vi "FRA-GRAPHs.vi"() -> ()   [LabVIEW 2014]
panel:
  in  "Waveform Graph":dbl[][](graph)=[[755.8497899944483, 657.3694630192037, 604.2075862163476, 553.4051094764117, 501.397888353343, 457.9831143953616, 522.5385383457407, 449.43840743756704, 491.0669063418323, 427.9053041861322, 472.8329741058286, 734.0752884613231, 754.8685930222813, 867.8139215972071, 764.1663113926469, 1052.3750959044867, 370.47956063576765, -5454.671583974405, 5956.812472120322, 3291.774216244163, 2978.0635239759176, 24470.64307332704, 24011.616955981375, 4002.6341189398554, 10685.523439025172, -1848.0447542106147, -644.1201502824483, 14733.80660145546, 35622.61812955256, 14965.266379348848, -30861.486423716706, 1459.6554322016723, -3196.3540839642674, 44188.99982358876, 45267.97553031476, 142706.1244173352, 53308.369203099464, -27391.526865018615, 183165.8872198102, -87308.9518464976, -120174.13920583515, 26604.096776415798, -493090.5307564318, 366117.10634527745, 543287.8874074903, -2290216.410117346, 1383746.3098287373, -841011.6581585368, -5069703.915509953], [12809.615219888727, 14640.640733060218, 16941.76975803665, 19632.39614327407, 22689.40920736704, 26187.18921639577, 30309.16414071273, 34780.24689799575, 40104.042390733164, 46225.486449506556, 53380.910426141934, 61315.525497053044, 70619.11169429292, 81129.69423706258, 92930.20554962437, 108052.78250593715, 123395.3276070273, 140233.9841683997, 162922.75157704714, 186591.72916940713, 218818.8824622036, 258336.1742390314, 284712.0097348884, 343587.40279145545, 384547.7548524852, 446876.68934418727, 533817.0452653471, 574035.5265669021, 740382.0640486595, 782382.9290463354, 916411.7746495624, 1020043.1012773687, 1177943.8671532222, 1318356.8890459158, 1599847.9327251778, 1898494.8612490473, 2005049.6933289415, 2218375.615595672, 2583265.3759603477, 3314305.664543704, 3723239.9116652273, 3990185.291575476, 5157765.897783338, 6377825.583902332, 7109284.559228457, 7483606.852740063, 6764537.148171906, 8811618.918211825, 7889126.237846744]]
  in  "Embedded Exe File":path=path "C:/Program Files/Metrohm Autolab/Autolab SDK 1.11/Hardware Setup Files/Adk.x"
  in  "Hardware Setup File":path=path "C:/Program Files/Metrohm Autolab/Autolab SDK 1.11/Hardware Setup Files/PGSTAT204/HardwareSetup.FRA32M.xml"
  in  "Nyquist":cluster{"Y":dbl[], "Y":dbl[]}[](graph)=[{"Y"=[717.4280419440639, 630.543336914633, 276.13049349252043, 1527.9648078341734, 778.7768911898802, -291.41103101988267, -1612.0992001939794, 22.840057454333408, 1766.9812060547838, 8705.573471549324, 61236.31899944996, 41607.235560112415, -11965.09300359767, -54468.84323488098, -210423.9025805467, -145222.68442226195, -104224.6172046195, -882870.4962035925, -502347.415485765, 445617.4744314733, 844265.0047461819, 230117.41559005968, -5144686.463770501, 3377559.916366239, 760509.6570473239, -2783991.8925627726, -1525489.689481452, -580636.4171269443, -794981.0784450348, -629094.5737383832, 1569220.258276646, 2825094.75316701, -1225387.2369710647, 113038.50874330386, -1737678.8550673486, 2992063.776927379, 992229.8811721486, 697881.8098522659, -271929.5901276921, -405193.6035110828, -584504.1041071352, 281262243.8893397, 896697484.8427294, -3273278095.7459807, -1350528375.109321, -7708436.093934186, -284016460.50012374, 1145108312.0465887, 1142034855.4732878], "Y"=[12713.490643849475, 16953.413875405506, 22664.767511323378, 30002.543878853052, 41476.30921506156, 54131.11924532798, 69659.62711739466, 93529.05430958046, 123123.69703312324, 218325.18626084126, 255444.3461274739, 194329.90284509392, 360601.74410314637, 537325.4921504976, 908162.746666654, 700008.1844468658, 1892074.040937823, 1563196.9541199794, 1851552.1342195985, 1760315.7277772645, 5099811.190634446, 2137795.767885032, 7725112.17693712, 3539552.0737207234, -6739223.001892976, -2251908.9120111996, -1789261.3987910943, 371509.23793097417, -72947.4350052079, 476875.5717505661, -1987000.3684945928, 4009293.059150154, 745260.0910446028, 1782107.0217877845, 1390223.1154664257, -436096.05494870833, 564131.9933859911, -622032.6124273272, 230091.1169243968, 3296653.446846964, 1434127.4994983494, 443672969.8487906, 1136000447.5621486, -1620943047.8641806, 505532133.16527915, 106057424.24216986, 4136536.231060236, 452143152.52999854, -123984503.52389096]}]
  in  "Bode phase":cluster{"Y":dbl[], "Y":dbl[]}[](graph)=[{"Y"=[100000.0, 75431.0, 56899.0, 42919.0, 32375.0, 24421.0, 18421.0, 13895.0, 10481.0, 7906.0, 5963.6, 4498.4, 3393.2, 2559.5, 1930.7, 1456.3, 1098.5, 828.64, 625.06, 471.49, 355.65, 268.27, 202.36, 152.64, 115.14000000000001, 86.851, 65.513, 49.417, 37.276, 28.117999999999995, 21.21, 15.999, 12.068, 9.103, 6.8665, 5.1795, 3.9069, 2.9471, 2.223, 1.6768, 1.2649, 0.9541, 0.71969, 0.54287, 0.40949, 0.30888, 0.233, 0.17575, 0.13257], "Y"=[86.77019859731325, 87.86999670170376, 89.30198581786577, 87.08456839663077, 88.92431638034876, 90.30844477483437, 91.3257319868692, 89.98600821018007, 89.17778934178514, 87.71657807960655, 76.51918215761853, 77.91507755936605, 91.9004287070616, 95.78831727337736, 103.04539451344091, 101.72024419185205, 93.15294303665505, 119.45711812667577, 105.17959047331752, 75.79421505865395, 80.60003568234677, 83.85620243872248, 123.66239108492334, 46.341567216211935, -83.56150902213479, -141.03137735157222, -130.4502686850989, 147.38762267357188, -174.75722298739544, 142.8366068171442, -51.700321013608495, 54.83007302178133, 148.6927302048697, 86.37060825361425, 141.33858273127964, -8.292521437931114, 29.62038195448254, -41.711101426708225, 139.76402867620763, 97.00711329520782, 112.17422406228579, 57.627736270324036, 51.71434155129174, -153.6551655871953, 159.4780326051847, 94.1570460820148, 179.16557895463174, 21.546461133036427, -6.196024073654414]}]
  in  "Bode Z":cluster{"Y":dbl[], "Y":dbl[]}[](graph)=[{"Y"=[100000.0, 75431.0, 56899.0, 42919.0, 32375.0, 24421.0, 18421.0, 13895.0, 10481.0, 7906.0, 5963.6, 4498.4, 3393.2, 2559.5, 1930.7, 1456.3, 1098.5, 828.64, 625.06, 471.49, 355.65, 268.27, 202.36, 152.64, 115.14000000000001, 86.851, 65.513, 49.417, 37.276, 28.117999999999995, 21.21, 15.999, 12.068, 9.103, 6.8665, 5.1795, 3.9069, 2.9471, 2.223, 1.6768, 1.2649, 0.9541, 0.71969, 0.54287, 0.40949, 0.30888, 0.233, 0.17575, 0.13257], "Y"=[12733.716949367761, 16965.135629593988, 22666.449532111907, 30041.426658141296, 41483.61989447946, 54131.90363492603, 69678.27863807869, 93529.05709838346, 123136.37559099615, 218498.6818388147, 262681.74800144584, 198734.1772084971, 360800.1958159333, 540079.1973387982, 932221.9656339088, 714913.3418557841, 1894942.4654121383, 1795284.1085568487, 1918488.5278724963, 1815843.1636511688, 5169222.144419738, 2150145.290473414, 9281441.534415092, 4892477.886636238, 6781998.349137636, 3580740.7900950764, 2351292.2289494514, 689316.8812397299, 798320.8899681065, 789411.3589501404, 2531920.749822844, 4904649.956777891, 1434219.8171254608, 1785688.4223078329, 2225364.7148558246, 3023677.4653297197, 1141387.3326143706, 934860.1988777999, 356212.89150525007, 3321461.395972301, 1548666.1139624233, 525313386.4771697, 1447260652.4688907, 3652643680.4744115, 1442043560.2429147, 106337186.45844391, 284046582.0371885, 1231140315.600928, 1148745301.7226923]}]
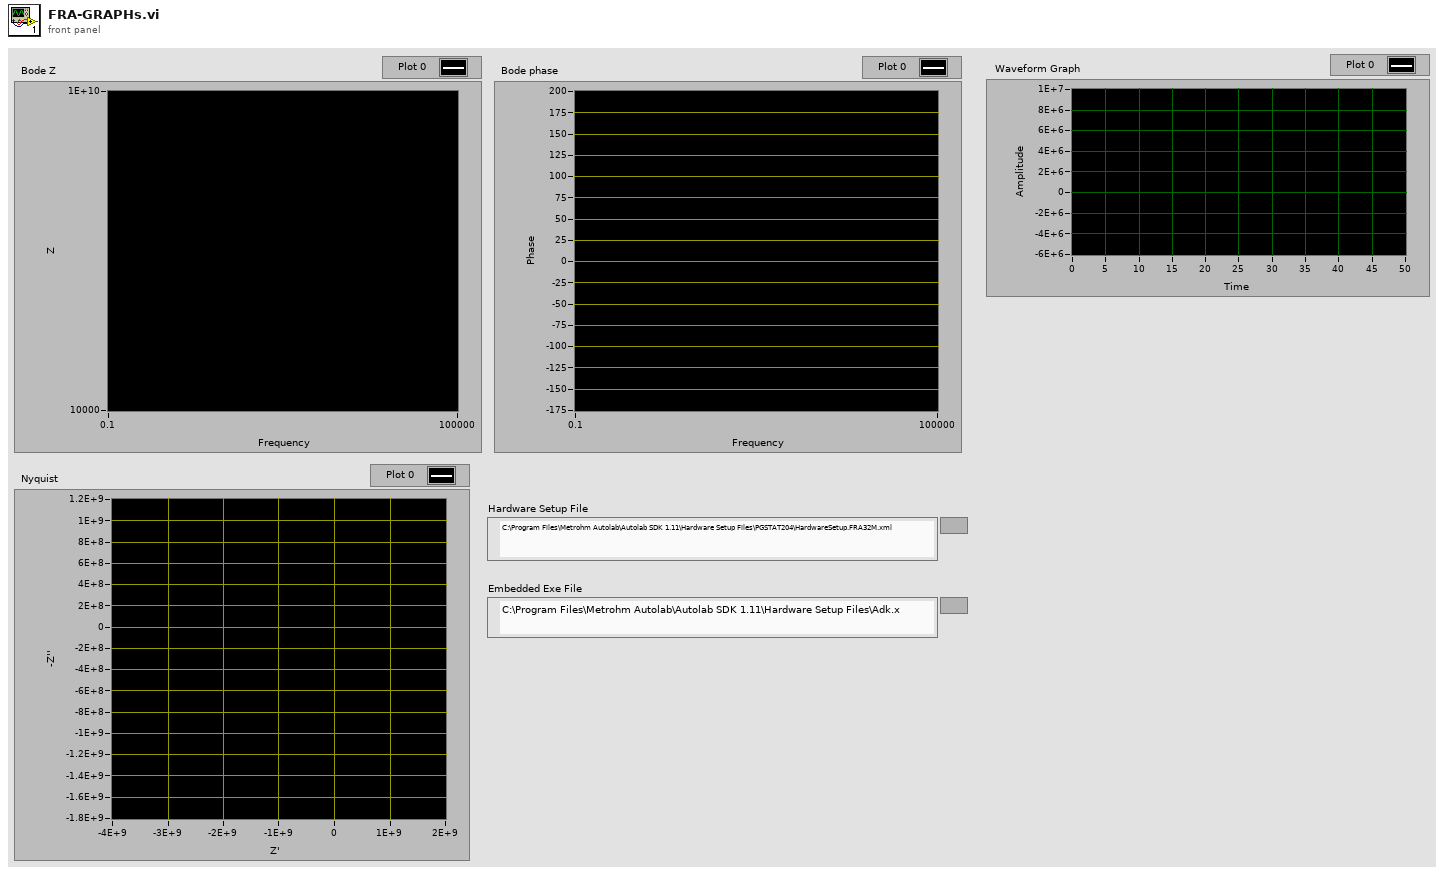
[diagram p1: front panel]
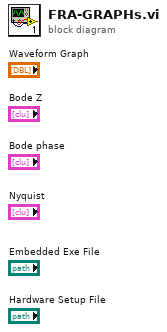
[diagram p0: block diagram]
diagram:
